vi "步骤数组元素入列队.vi"(8 "错误输入（无错误）":errorcluster, 9 "队列":refnum<queue>, 10 "添加的数组":string[][](array[string]), 11 "名称（未命名）":string) -> (0 "错误输出":errorcluster, 1 "队列输出":refnum<queue>, 3 "簇数组":cluster{"添加的数组 2":string[]}[](array[cluster]))   [LabVIEW 2016]
panel:
  out "队列中元素数量":i32
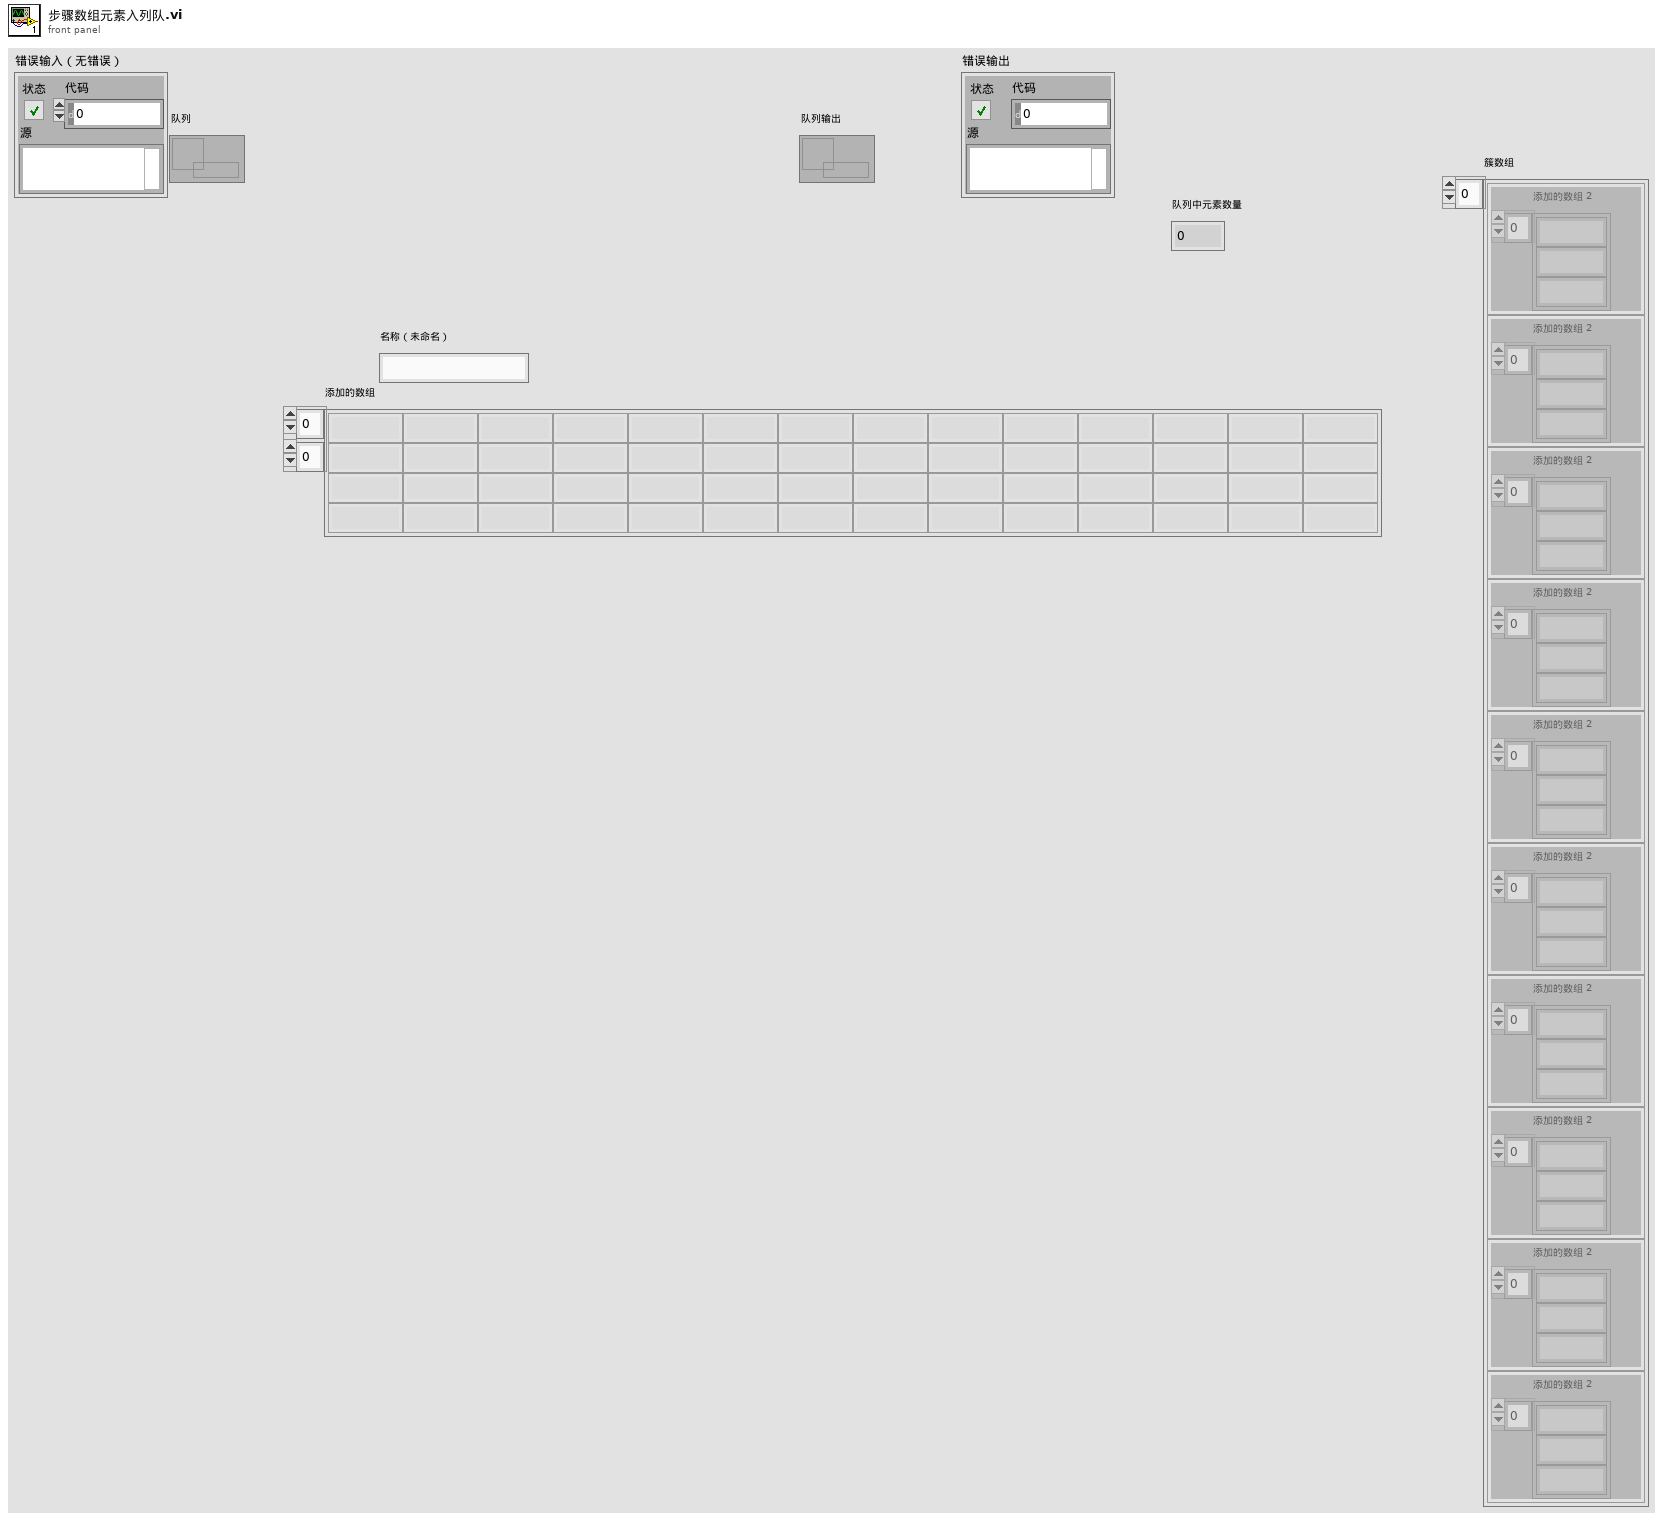
[diagram p1: front panel]
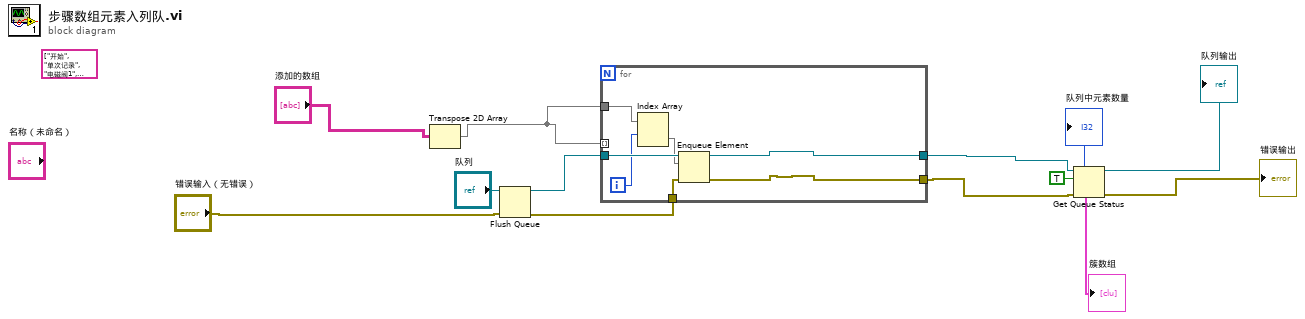
[diagram p0: block diagram]
diagram:
  (unwired) string[] ["开始", "单次记录", "电磁阀1", "报警器开", "气泵1、2", "Set Valve Position", "等待", "暂停", "跳转事件"] ("添加的数组 2")
  n1 = Transpose 2D Array(2D array="添加的数组") -> (transposed array=w10:string[][])
  n2 = Flush Queue(queue="队列", error in (no error)="错误输入（无错误）") -> (queue out=w12:refnum<queue>, error out=w11:errorcluster)  [unwired: 1 out]
  n3 = for {
    tunnel: w10 -> [_] mode=indexing
    tunnel: w12 -> [w20]
    tunnel: w11 -> [w19]
    tunnel: [w15] -> w7
    tunnel: [w14] -> w6
    tunnel: w10 -> [w18]
    i -> [w17]
    n4 = Index Array(array=w18, index (row)=w17) -> (element=w16:string[])  [unwired: 1 in]
    n5 = Enqueue Element(queue=w20, element=w16, error in (no error)=w19) -> (queue out=w15:refnum<queue>, error out=w14:errorcluster)  [unwired: 1 in, 1 out]
  }
  n6 = Get Queue Status(queue=w7, return elements? (F)=TRUE ("返回元素？(F)"), error in (no error)=w6) -> (queue out=→"队列输出":refnum<queue>, error out=→"错误输出":errorcluster, # elements in queue=→"队列中元素数量":i32, elements=→"簇数组":cluster{"添加的数组 2":string[]}[])  [unwired: 4 out]
